vi "Find Nodes.vi"(11 "Array in":string[][](array[string])) -> (3 "Array out":cluster{i32, i32}[](array[cluster]))   [LabVIEW 2021]
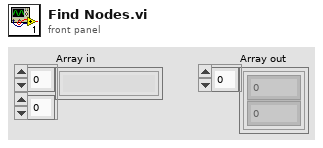
[diagram p1: front panel]
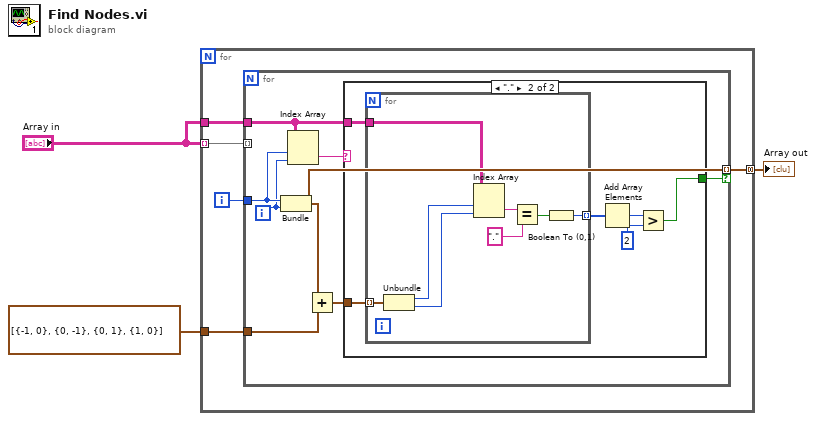
[diagram p0: block diagram]
diagram:
  n1 = for {
    tunnel: "Array in" -> [w8] mode=indexing
    tunnel: cluster{i32, i32}[] [{-1, 0}, {0, -1}, {0, 1}, {1, 0}] -> [w6]
    tunnel: "Array in" -> [w5]
    tunnel: [w4] -> w2 mode=concatenating
    i -> [w7]
    n2 = for {
      tunnel: w8 -> [_] mode=indexing
      tunnel: w7 -> [w12]
      tunnel: w6 -> [w16]
      tunnel: w5 -> [w10]
      tunnel: [w14] -> w4 mode=indexing if=w13
      i -> [w11]
      n3 = Bundle(w12, w11) -> (w14:cluster{i32, i32})  [unwired: 1 in]
      n4 = Index Array(array=w10, index (row)=w12, index (col)=w11) -> (element=w9:string)
      n5 = Add(x=w14, y=w16) -> (x+y=w15:cluster{i32, i32}[])
      n6 = case shown="\".\"" w9 {
        tunnel: w15 -> [_ w22]
        tunnel: [_ w18] -> w13
        tunnel: w10 -> [_ w17]
        frame Default {
        }
        frame "." {
          n7 = for {
            tunnel: w17 -> [w30]
            tunnel: w22 -> [w29] mode=indexing
            tunnel: [w23] -> w21 mode=indexing
            n8 = Unbundle(w29) -> (w28:i32, w27:i32)
            n9 = Index Array(array=w30, index (row)=w28, index (col)=w27) -> (element=w26:string)
            n10 = Equal?(x=w26, y=".") -> (x = y?=w24:bool)
            n11 = Boolean To (0,1)(Boolean=w24) -> (0, 1=w23:i16)
          }
          n12 = Add Array Elements(numeric array=w21) -> (sum=w20:i16)
          n13 = Greater?(x=w20, y=2) -> (0:w18:bool)
        }
      }
    }
  }
  "Array out" <- w2
